vi "Control Panel Controller.vi"(8 "error in":errorcluster) -> ()   [LabVIEW 2019]
doc: "This VI executes continuously carrying out the current operation and responding to updates or new operations. It will often contain the timing or control code that is difficult to place directly in TeleOp. This VI generally opens all sensors and motors and isolates the rest of the robot code from knowing how the operations are carried out."
uses:
  <vilib>/Rock Robotics/WPI/Framework/Completion Status.ctl
  Control Panel Setpoints.ctl
  Control Panel Operations.ctl
  <vilib>/Rock Robotics/SystemInterfaces/i2clib/i2c_bus.ctl
  <vilib>/Rock Robotics/WPI/ThirdParty/Phoenix-LabVIEW/Motor Controller/Controls/CTRE_Phoenix_MotorControl_ControlMode.ctl
  <vilib>/Rock Robotics/Network Tables/NT Write Boolean.vi
panel:
  out "Matched Color Name 2":string
  out "Match Confidence 2":dbl
  out "Measured Color 2":cluster{"R":dbl, "G":dbl, "B":dbl}
  out "error out 2":errorcluster
  out "Proximity 2":u16(graph)
  out "Color 2":u32(colorbox)
  out "Matched Color Name":string
  out "Match Confidence":dbl
  out "Measured Color":cluster{"R":dbl, "G":dbl, "B":dbl}
  out "error out":errorcluster
  out "Proximity":u16(graph)
  out "Color":u32(colorbox)
  in  "I2C Bus":T1
  in  "Blue Calibration":cluster{"R":dbl, "G":dbl, "B":dbl}={"R"=0.143, "G"=0.427, "B"=0.429}
  in  "Green Calibration":cluster{"R":dbl, "G":dbl, "B":dbl}={"R"=0.197, "G"=0.561, "B"=0.24}
  in  "Red Calibration":cluster{"R":dbl, "G":dbl, "B":dbl}={"R"=0.561, "G"=0.323, "B"=0.114}
  in  "Yellow Calibration":cluster{"R":dbl, "G":dbl, "B":dbl}={"R"=0.361, "G"=0.524, "B"=0.113}
  in  "Interactive Values":T2
  out "Current\nCmd":string
  in  "Buttons":cluster{"Execute Cmd":bool, "Abort Cmd":bool}
  out "Command Timing":cluster{"Start Time (ms)":u32, "Iterations":i32}
  out "Status":T4
  # "Tip: It may be helpful to observe inputs and sensor values.\nYou may also want to display tuning or debugging controls."
  # "Interactive Command: You may fill in the settings for a command\nand schedule it with the Execute button. You can observe and abort\nany command while fine tuning the code for the controller."
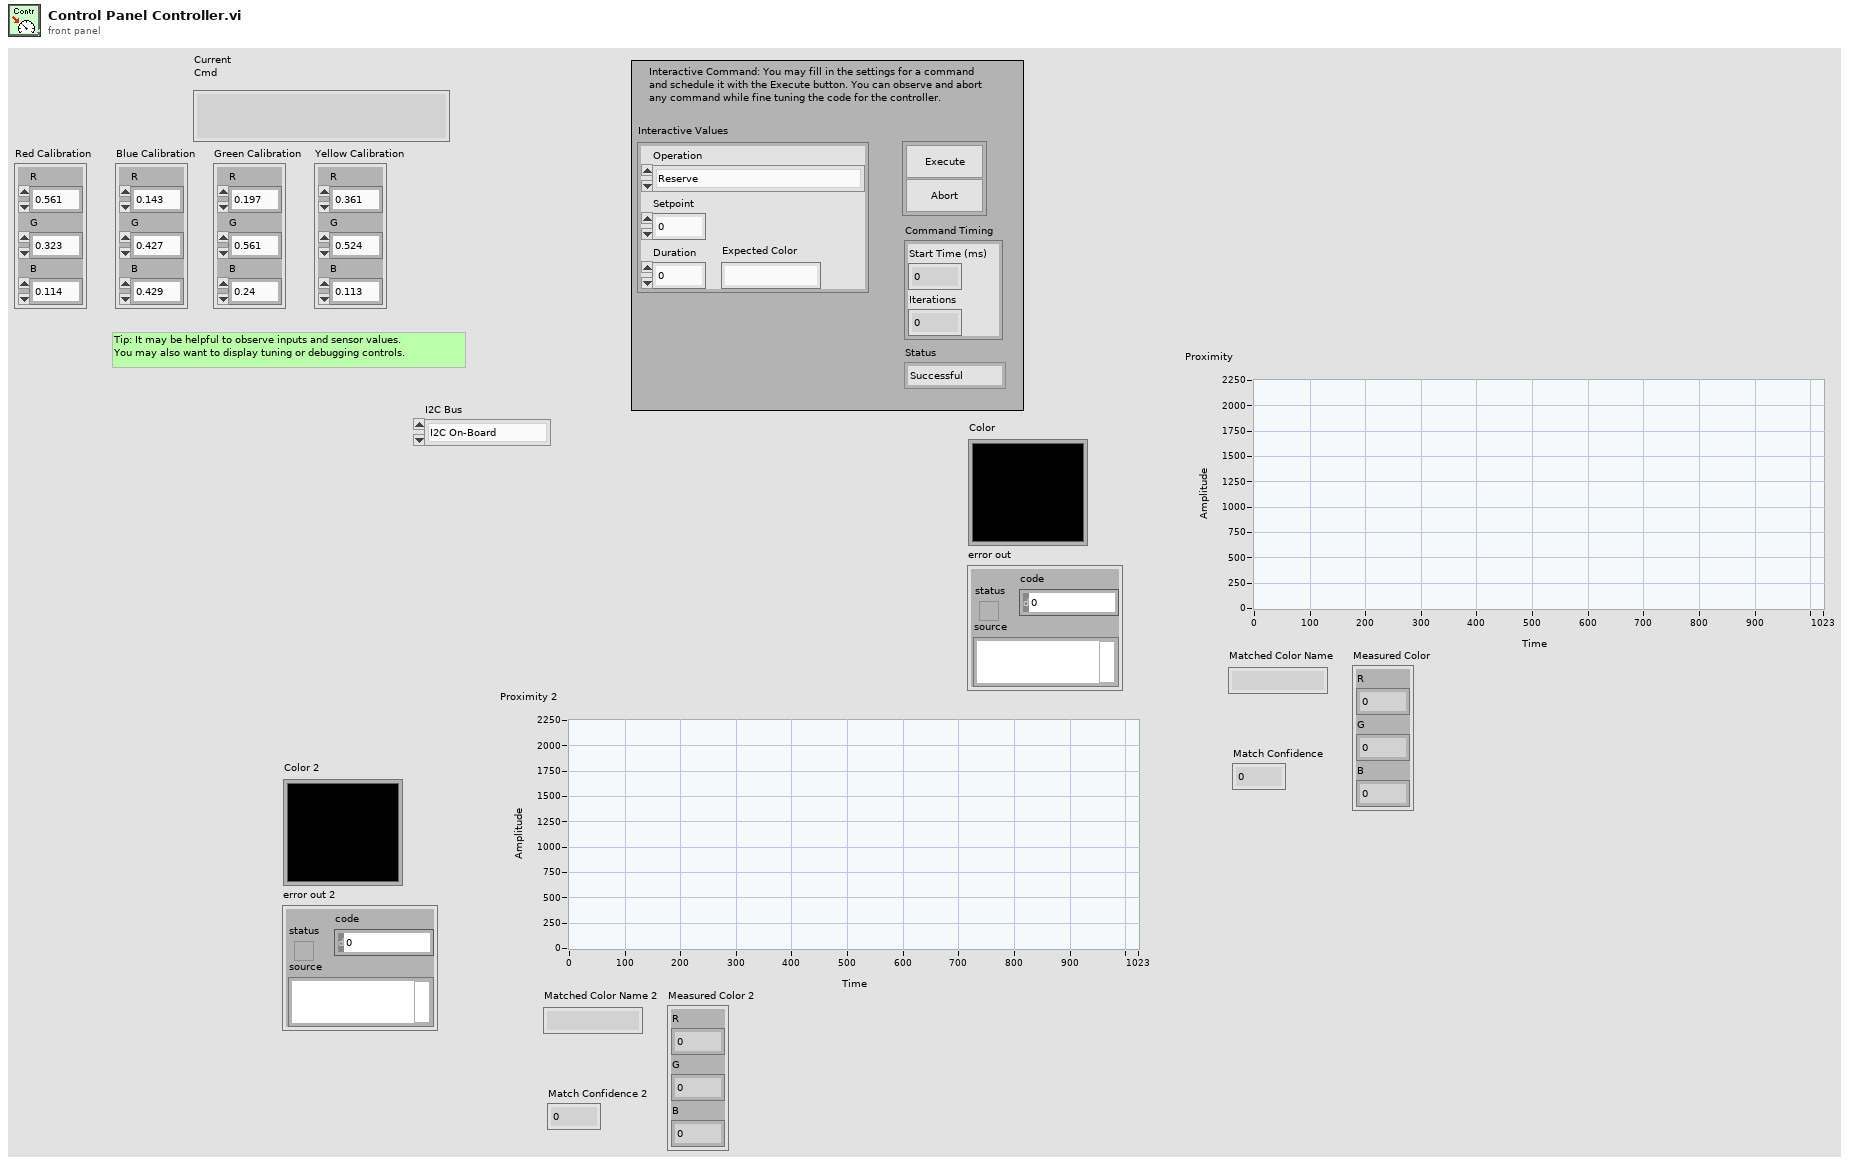
[diagram p1: front panel]
types:
  T1 = typedef "i2c_bus.ctl" = enum16{"I2C On-Board", "I2C MXP", "Invalid"}
  T2 = typedef "Control Panel Setpoints.ctl" = cluster{"Operation":T3, "Setpoint":dbl, "Duration":dbl, "Expected Color":string}
  T3 = typedef "Control Panel Operations.ctl" = enum16{"Reserve", "Read Current", "Immediate", "Rotation control", "Color control"}
  T4 = typedef "Completion Status.ctl" = enum16{"Successful", "Aborted", "Incomplete"}
  T5 = typedef "Color Sensor V3 DevRef.ctl" = cluster{"I2CDevRef":T6}
  T6 = typedef "WPI_I2CDevRef.ctl" = cluster{"DevStatus":errorcluster, "Device Address":u8, "Handle":i32, "I2C Bus":T1}
  T7 = typedef "CTRE_Phoenix_MotorControl_ControlMode.ctl" = u16
  T8 = typedef "Command Status Info.ctl" = cluster{"Name":string, "Status":T4, "notifier out":T9}
  T9 = typedef "Completion Notifier.ctl" = refnum<notifier>
  T10 = cluster{"Current Command":T2, "Command Timing":cluster{"Start Time (ms)":u32, "Iterations":i32}, "Command Arguments":cluster{"Command Info":T8, "Description":string, "Default Command":T2, "queue out":refnum<queue>, "Subsystem Name":string}}
  T11 = typedef "WPI_MotorControlDeviceRef.ctl" = cluster{"DeviceStatus":errorcluster, "Type":T12, "PWM":cluster{"PWM Channel":T13, "DeadBand":T14}, "CAN":cluster{"Device Number":u8, "SetOutput VI Ref":variant, "GetOutput VI Ref":variant, "Enable VI Ref":variant, "Disable VI Ref":variant, "Data":variant}, "Invert":bool, "DIO PWM":cluster{"PWM \"Enable\" Channel":T13, "DIOChannel":T15, "PWM Rate":dbl}}
  T12 = typedef "WPI_MotorControlType.ctl" = enum16{"PWM", "CAN", "DIO PWM"}
  T13 = typedef "FPGA_DIOPWMChannel.ctl" = enum8{"PWM 0", "PWM 1", "PWM 2", "PWM 3", "PWM 4", "PWM 5", "PWM 6", "PWM 7", "PWM 8", "PWM 9", "PWM MXP 0", "PWM MXP 1", "PWM MXP 2", "PWM MXP 3", "PWM MXP 4", "PWM MXP 5", "PWM MXP 6", "PWM MXP 7", "PWM MXP 8", "PWM MXP 9", "Invalid"}
  T14 = typedef "WPI_PWMDeadband.ctl" = cluster{"Name":string, "maxPositivePwm":i32, "minPositivePwm":i32, "centerPwm":i32, "maxNegativePwm":i32, "minNegativePwm":i32, "angularRange":u16}
  T15 = typedef "FPGA_DIOChannel.ctl" = enum8{"DIO 0", "DIO 1", "DIO 2", "DIO 3", "DIO 4", "DIO 5", "DIO 6", "DIO 7", "DIO 8", "DIO 9", "DIO MXP 0", "DIO MXP 1", "DIO MXP 2", "DIO MXP 3", "DIO MXP 4", "DIO MXP 5", "DIO MXP 6", "DIO MXP 7", "DIO MXP 8", "DIO MXP 9", "DIO MXP 10", "DIO MXP 11", "DIO MXP 12", "DIO MXP 13", "DIO MXP 14", "DIO MXP 15", "SPI Port CS1", "SPI Port CS2", "SPI Port CS3", "SPI Port MISO", "SPI Port MOSI", "Invalid"}
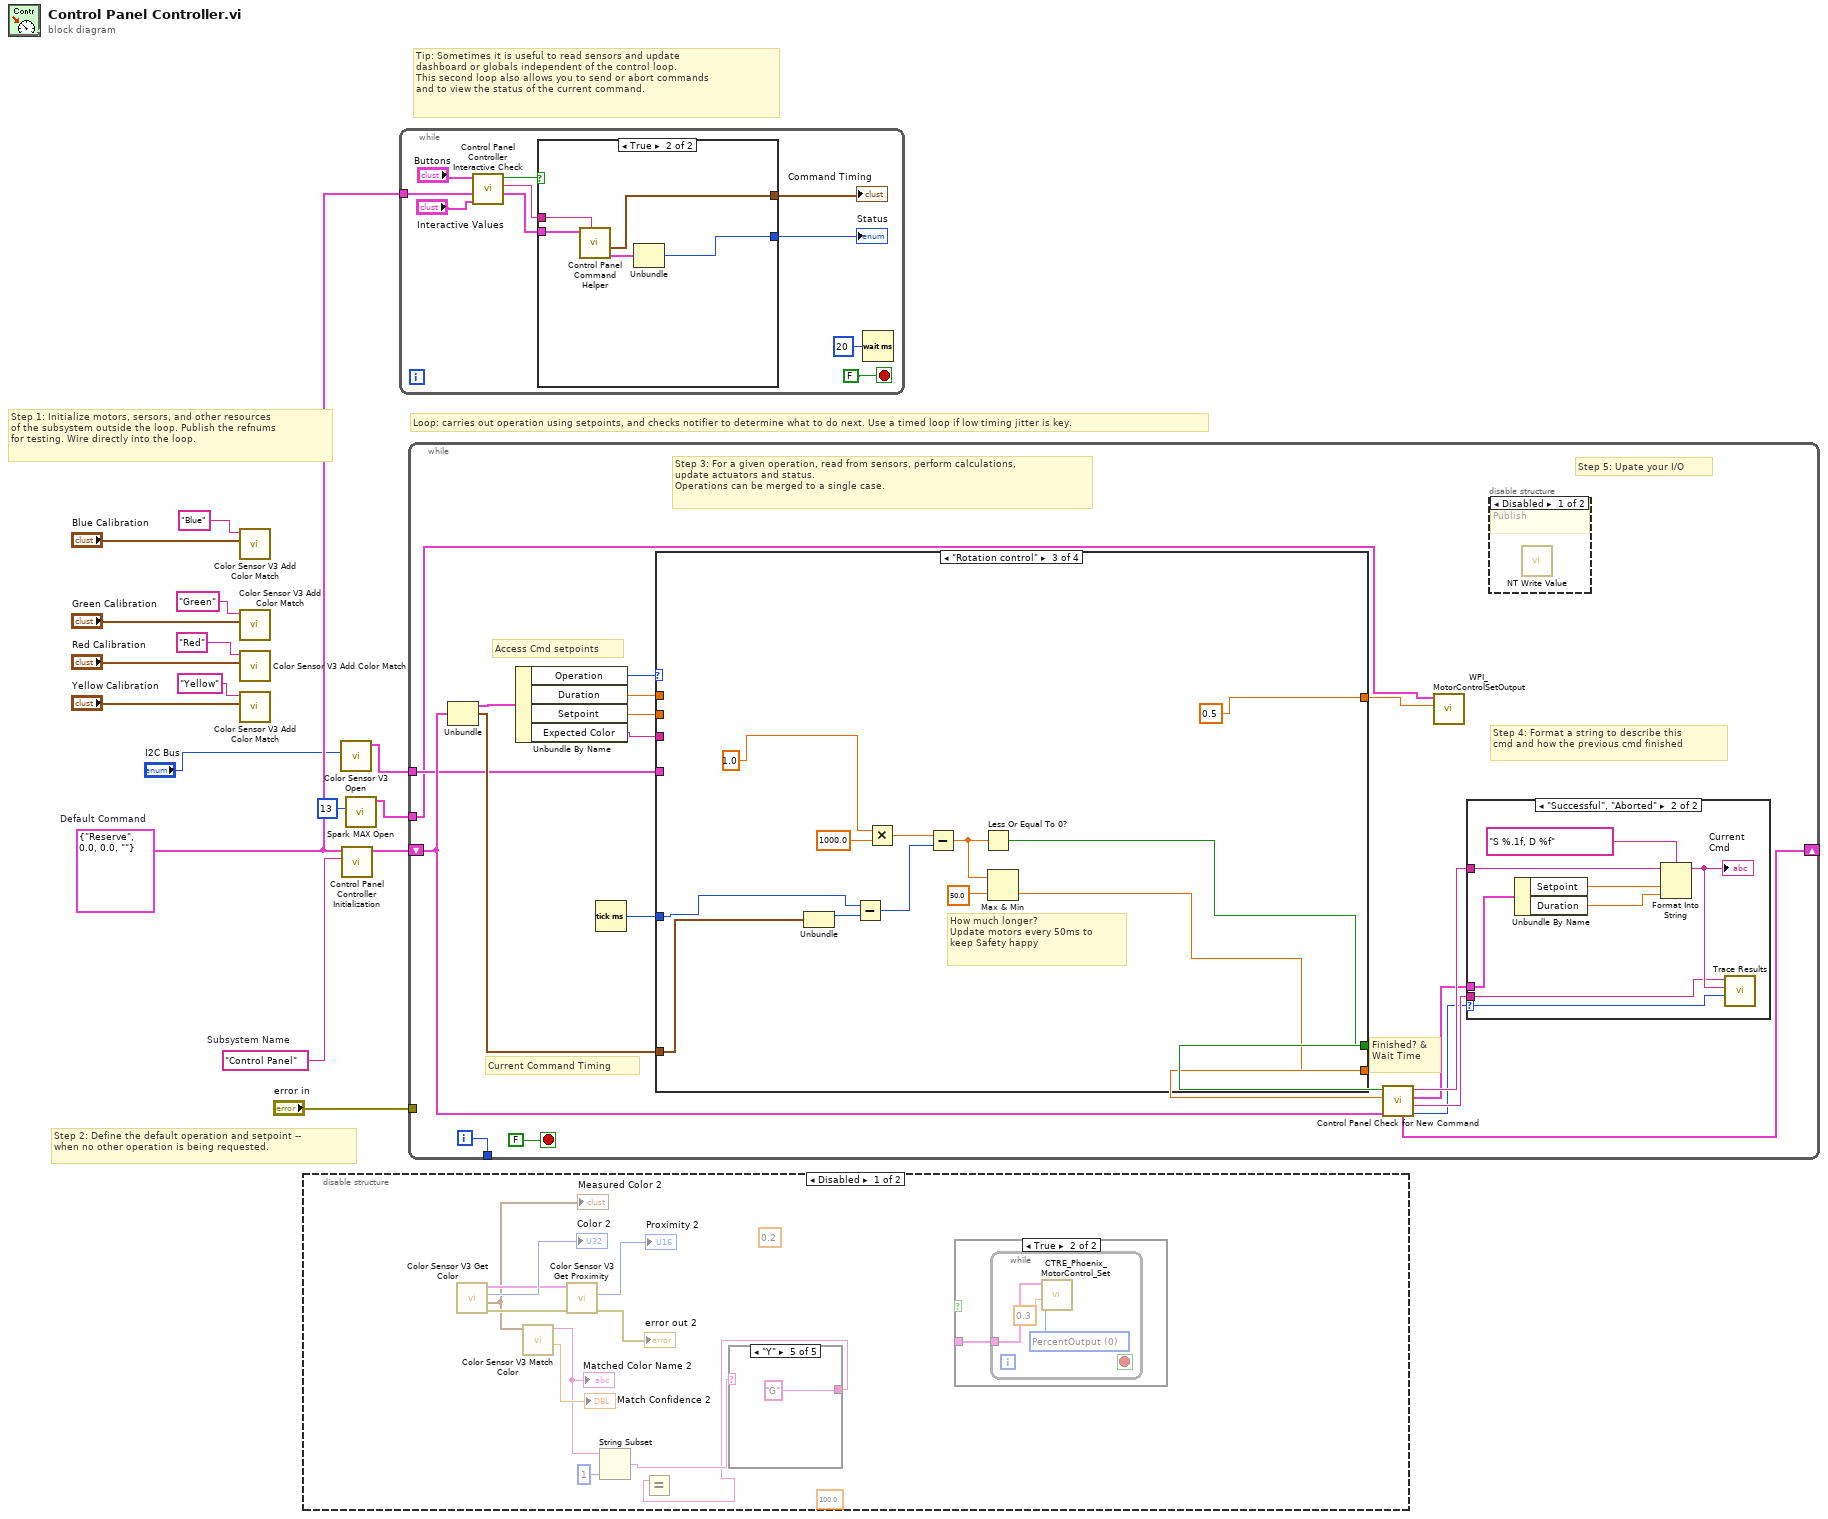
[diagram p0: block diagram]
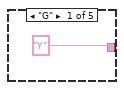
[diagram p3: hidden frame]
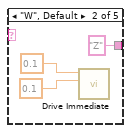
[diagram p4: hidden frame]
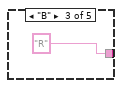
[diagram p5: hidden frame]
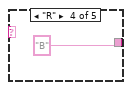
[diagram p6: hidden frame]
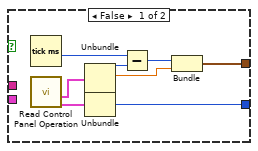
[diagram p8: hidden frame]
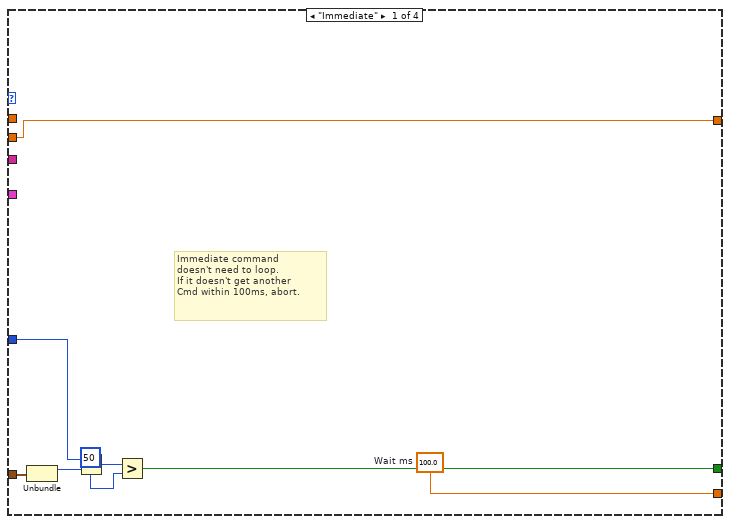
[diagram p11: hidden frame]
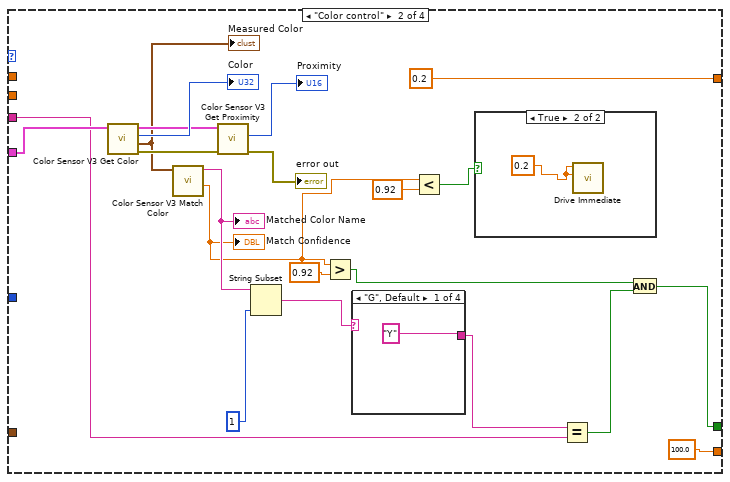
[diagram p12: hidden frame]
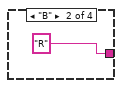
[diagram p13: hidden frame]
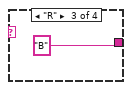
[diagram p14: hidden frame]
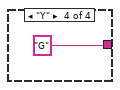
[diagram p15: hidden frame]
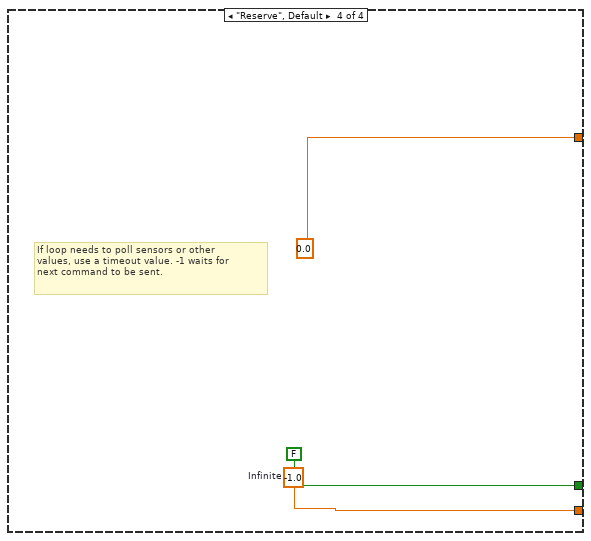
[diagram p17: hidden frame]
diagram:
  w13 = T2 {"Operation"=enum."Reserve", "Setpoint"=0.0, "Duration"=0.0, "Expected Color"=""}  # Default Command
  w14 = "Control Panel"  # Subsystem Name
  # "Tip: Sometimes it is useful to read sensors and update\ndashboard or globals independent of the control loop.\nThis second loop also allows you to send or abort commands\nand to view the status of the current command."
  # "Step 2: Define the default operation and setpoint --\nwhen no other operation is being requested."
  # "Step 1: Initialize motors, sersors, and other resources\nof the subsystem outside the loop. Publish the refnums\nfor testing. Wire directly into the loop."
  # "Loop: carries out operation using setpoints, and checks notifier to determine what to do next. Use a timed loop if low timing jitter is key."
  n1 = call <vilib>:"Color Sensor V3 Add Color Match.vi"("Color"="Blue Calibration", "Name"="Blue") -> ()  [unwired: 10 in]
  n2 = call <vilib>:"Color Sensor V3 Add Color Match.vi"("Color"="Green Calibration", "Name"="Green") -> ()  [unwired: 10 in]
  n3 = call <vilib>:"Color Sensor V3 Add Color Match.vi"("Color"="Red Calibration", "Name"="Red") -> ()  [unwired: 10 in]
  n4 = call <vilib>:"Color Sensor V3 Add Color Match.vi"("Color"="Yellow Calibration", "Name"="Yellow") -> ()  [unwired: 10 in]
  n5 = disable-structure shown="Disabled" {
    frame Disabled {
      w21 = 0.2
      (unwired) 100.0 ("Infinite")
      n6 = call <vilib>:"Color Sensor V3 Get Color.vi"() -> ("error out"=w30:errorcluster, "Normalized Color"=w27:cluster{"R":dbl, "G":dbl, "B":dbl}, "Color"=→"Color 2":u32, "ColorSensorDevRef out"=w29:T5, "ColorSensorDevRef"=w24:T5)  [unwired: 7 in]
      "Measured Color 2" <- w27
      n7 = call <vilib>:"Color Sensor V3 Match Color.vi"("Measured Color"=w27) -> ("Confidence"=→"Match Confidence 2":dbl, "Matched Color Name"=w20:string)  [unwired: 8 in, 1 out]
      "Matched Color Name 2" <- w20
      n8 = call <vilib>:"Color Sensor V3 Get Proximity.vi"("error in (no error)"=w30, "ColorSensorDevRef"=w29) -> ("error out"=→"error out 2":errorcluster, "Proximity"=→"Proximity 2":u16)  [unwired: 7 in, 1 out]
      n9 = String Subset(string=w20, length (rest)=1 ("length (rest)")) -> (substring=w18:string)  [unwired: 1 in]
      n10 = case shown="\"Y\"" w18 {
        tunnel: ["Y" "Z" "R" "B" "G"] -> w17
        frame "G" {
        }
        frame "W", Default {
          n11 = call "Drive Immediate.vi"("Right Setpoint"=0.1, "Left Setpoint"=0.1) -> ()  [unwired: 9 in, 1 out]
        }
        frame "B" {
        }
        frame "R" {
        }
        frame "Y" {
        }
      }
      n12 = Equal?(x=w17) -> (y=w23:string, x = y?=w22:bool)
      n13 = case shown="True" {
        selector: _ -> [_ _]
        tunnel: _ -> [_ w32]
        frame False {
        }
        frame True {
          n14 = while {
            tunnel: w32 -> [w35]
            stop <- _ stop-if-true
            w34 = T7 0 items=["PercentOutput"=0, "Position"=1, "Velocity"=2, "Current"=3, "Follower"=5, "MotionProfile"=6, "MotionMagic"=7, "MotionProfileArc"=10, "Disabled"=15] ("Control Mode")
            n15 = call <vilib>:"CTRE_Phoenix_MotorControl_Set.vi"("Output"=0.3, "Control Mode"=w34, "PhoenixMotorControlDevRef"=w35) -> ()  [unwired: 7 in, 2 out]
          }
        }
      }
    }
    frame Enabled {
    }
  }
  n16 = call <vilib>:"Color Sensor V3 Open.vi"("I2C Bus"="I2C Bus") -> ("ColorSensorDevRef"=w3:T5)  [unwired: 9 in, 1 out]
  n17 = call "Control Panel Controller Initialization.vi"("Subsystem Name"=w14, "Default Command"=w13) -> ("Current Command"=w15:T10)  [unwired: 9 in]
  n18 = call <vilib>:"Spark MAX Open.vi"("Device Number"=u8 13) -> ("MotorControlDeviceRef"=w1:T11)  [unwired: 9 in, 1 out]
  n19 = while {
    tunnel: w13 -> [w49]
    stop <- FALSE stop-if-true
    n20 = call "Control Panel Controller Interactive Check.vi"("Interactive Command in"="Interactive Values", "Default Command"=w49, "Buttons"="Buttons") -> ("Interactive Command out"=w46:T2, "Trace String"=w47:string, "Schedule"=w48:bool)  [unwired: 6 in]
    n21 = case shown="True" w48 {
      tunnel: [w60 w65] -> w45
      tunnel: w46 -> [_ w63]
      tunnel: [w56 w61] -> w44
      tunnel: w47 -> [_ w64]
      frame False {
        n22 = Tick Count (ms)() -> (millisecond timer value=w55:u32)
        n23 = call "Read Control Panel Operation.vi"() -> ("Command Info"=w53:T8, "SubSystem Data"=w54:T2)  [unwired: 9 in, 1 out]
        n24 = Unbundle(w54) -> ("Operation"=w59:T3, "Setpoint"=w57:dbl)  [unwired: 2 out]
        n25 = Unbundle(w53) -> ("Status"=w60:T4)  [unwired: 2 out]
        n26 = Subtract(x=w55, y=w59) -> (x-y=w58:u32)
        n27 = Bundle(w58, "Setpoint"=w57) -> (w56:cluster{u32, "Setpoint":dbl})  [unwired: 1 in]
      }
      frame True {
        n28 = call "Control Panel Command Helper.vi"("Description"=w64, "SubSystem Data"=w63) -> ("Command Info Out"=w62:T8, "Command Timing"=w61:cluster{"Start Time (ms)":u32, "Iterations":i32})  [unwired: 7 in, 1 out]
        n29 = Unbundle(w62) -> ("Status"=w65:T4)  [unwired: 2 out]
      }
    }
    "Status" <- w45
    "Command Timing" <- w44
    n30 = Wait (ms)(milliseconds to wait=u32 20) -> ()  [unwired: 1 out]
  }
  n31 = while {
    shift-right: [w77] -> _
    shift-left: w15 -> [w70]
    tunnel: [w84] -> _
    tunnel: "error in" -> [_]
    tunnel: w3 -> [w68]
    tunnel: w1 -> [w66]
    i -> [w84]
    stop <- FALSE stop-if-true
    # "Step 5: Upate your I/O"
    # "Step 4: Format a string to describe this\ncmd and how the previous cmd finished"
    # "Current Command Timing"
    # "Access Cmd setpoints"
    # "Finished? &\nWait Time"
    # "Step 3: For a given operation, read from sensors, perform calculations,\nupdate actuators and status.\nOperations can be merged to a single case."
    n32 = Unbundle(w70) -> ("Current Command"=w83:T2, "Command Timing"=w79:cluster{"Start Time (ms)":u32, "Iterations":i32})  [unwired: 1 out]
    n33 = Unbundle By Name(w83) -> ("Operation"=w82:T3, "Duration"=w81:dbl, "Setpoint"=w78:dbl, "Expected Color"=w69:string)
    n34 = Tick Count (ms)() -> (millisecond timer value=w80:u32)
    n35 = case shown="\"Rotation control\"" w82 {
      tunnel: [w101 100.0 ("Infinite") w129 w142] -> w75
      tunnel: [w95 w107 w130 FALSE ("ignore previous (F)")] -> w76
      tunnel: w79 -> [w97 _ w131 _]
      tunnel: w81 -> [_ _ _ _]
      tunnel: w80 -> [w96 _ w132 _]
      tunnel: w78 -> [w94 _ _ _]
      tunnel: w69 -> [_ w115 _ _]
      tunnel: w68 -> [_ w116 _ _]
      tunnel: [w94 0.2 0.5 0.0] -> w67
      frame "Immediate" {
        w101 = 100.0  # Wait ms
        # "Immediate command\ndoesn't need to loop.\nIf it doesn't get another\nCmd within 100ms, abort."
        n36 = Unbundle(w97) -> ("Start Time (ms)"=w100:u32)  [unwired: 1 out]
        n37 = Subtract(x=w96, y=w100) -> (x-y=w99:u32)
        n38 = Greater?(x=w99, y=u8 50 ("Left Motor")) -> (0:w95:bool)
      }
      frame "Color control" {
        n39 = call <vilib>:"Color Sensor V3 Get Color.vi"("ColorSensorDevRef"=w116) -> ("error out"=w121:errorcluster, "Normalized Color"=w118:cluster{"R":dbl, "G":dbl, "B":dbl}, "Color"=→"Color":u32, "ColorSensorDevRef out"=w120:T5)  [unwired: 7 in]
        "Measured Color" <- w118
        n40 = call <vilib>:"Color Sensor V3 Match Color.vi"("Measured Color"=w118) -> ("Confidence"=w106:dbl, "Matched Color Name"=w112:string)  [unwired: 8 in, 1 out]
        "Match Confidence" <- w106
        "Matched Color Name" <- w112
        n41 = call <vilib>:"Color Sensor V3 Get Proximity.vi"("error in (no error)"=w121, "ColorSensorDevRef"=w120) -> ("error out"=→"error out":errorcluster, "Proximity"=→"Proximity":u16)  [unwired: 7 in, 1 out]
        n42 = String Subset(string=w112, length (rest)=1 ("length (rest)")) -> (substring=w103:string)  [unwired: 1 in]
        n43 = Greater?(x=w106, y=0.92) -> (0:w110:bool)
        n44 = case shown="\"G\", Default" w103 {
          tunnel: ["Y" "R" "B" "G"] -> w102
          frame "G", Default {
          }
          frame "B" {
          }
          frame "R" {
          }
          frame "Y" {
          }
        }
        n45 = Less?(x=w106, y=0.92) -> (x < y?=w104:bool)
        n46 = case shown="True" w104 {
          frame False {
          }
          frame True {
            w127 = 0.2
            n47 = call "Drive Immediate.vi"("Right Setpoint"=w127, "Left Setpoint"=w127) -> ()  [unwired: 9 in, 1 out]
          }
        }
        n48 = Equal?(x=w102, y=w115) -> (x = y?=w108:bool)
        n49 = And(x=w110, y=w108) -> (x .and. y?=w107:bool)
      }
      frame "Rotation control" {
        # "How much longer?\nUpdate motors every 50ms to\nkeep Safety happy"
        n50 = Unbundle(w131) -> ("Start Time (ms)"=w136:u32)  [unwired: 1 out]
        n51 = Subtract(x=w132, y=w136) -> (x-y=w139:u32)
        n52 = Multiply(x=1.0, y=1000.0) -> (x*y=w138:dbl)
        n53 = Subtract(x=w138, y=w139) -> (x-y=w135:dbl)
        n54 = Less Or Equal To 0?(x=w135) -> (x <= 0?=w130:bool)
        n55 = Max & Min(x=w135, y=50.0) -> (min(x,y)=w129:dbl)  [unwired: 1 out]
      }
      frame "Reserve", Default {
        w142 = -1.0  # Infinite
        # "If loop needs to poll sensors or other\nvalues, use a timeout value. -1 waits for\nnext command to be sent."
      }
    }
    n56 = call "Control Panel Check for New Command.vi"("Current Command"=w70, "Wait time (ms)"=w75, "Finished?"=w76) -> ("Completion"=w71:T4, "Subsystem Name"=w72:string, "Current Command"=w73:T2, "Initial Trace String"=w74:string, "NextCommand"=w77:T10)  [unwired: 4 in]
    n57 = call <vilib>:"WPI_MotorControlSetOutput.vi"("Output"=w67, "MotorControlDevRef"=w66) -> ()  [unwired: 7 in, 3 out]
    n58 = case shown="\"Successful\", \"Aborted\"" w71 {
      selector: w71 -> [_ w93]
      tunnel: w74 -> [_ w89]
      tunnel: w73 -> [_ w90]
      tunnel: w72 -> [_ w86]
      frame "Incomplete", Default {
        # "Continuing current command"
      }
      frame "Successful", "Aborted" {
        # "Report and setup for next command"
        n59 = Unbundle By Name(w90) -> ("Setpoint"=w92:dbl, "Duration"=w87:dbl)
        n60 = Format Into String(format string="S %.1f, D %f", initial string=w89, w92, w87) -> (resulting string=w88:string)  [unwired: 1 in, 1 out]
        "Current\nCmd" <- w88
        n61 = call <vilib>:"Trace Results.vi"("Status of previous command"=w93, "Description"=w88, "Subsystem"=w86) -> ()  [unwired: 9 in]
      }
    }
    n62 = disable-structure shown="Disabled" {
      frame Disabled {
        # "Publish"
        n63 = call-poly <vilib>:"NT Write Value.vi"() -> ()  [unwired: 11 in, 1 out]
      }
      frame Enabled {
      }
    }
  }
